vi "Update State Data.vi"(8 "error in (no error)":errorcluster, 9 "Data":variant, 10 "Argument":string, 11 "Window Action in":refnum<class "Window Action.lvclass">) -> (0 "error out":errorcluster, 3 "Window Action out":refnum<class "Window Action.lvclass">)   [LabVIEW 2020, in "MacroAssert.lvlib" / "Window Action.lvclass"]
uses:
  Window Action.lvclass
  Window Action Type.ctl
  Action Step/Action Step.lvclass
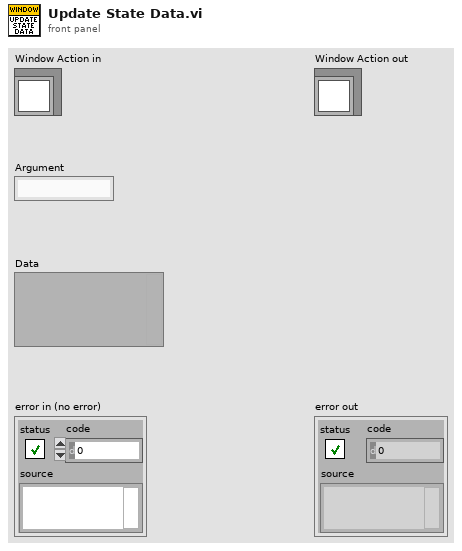
[diagram p1: front panel]
types:
  T1 = typedef "MacroAssert.lvlib/Window Action.lvclass/Window Action Type.ctl" = enum16{"Maximize Window", "Restore Window", "Minimize Window", "Close Window", "Bring Window to Front", "Send Window to Back"}
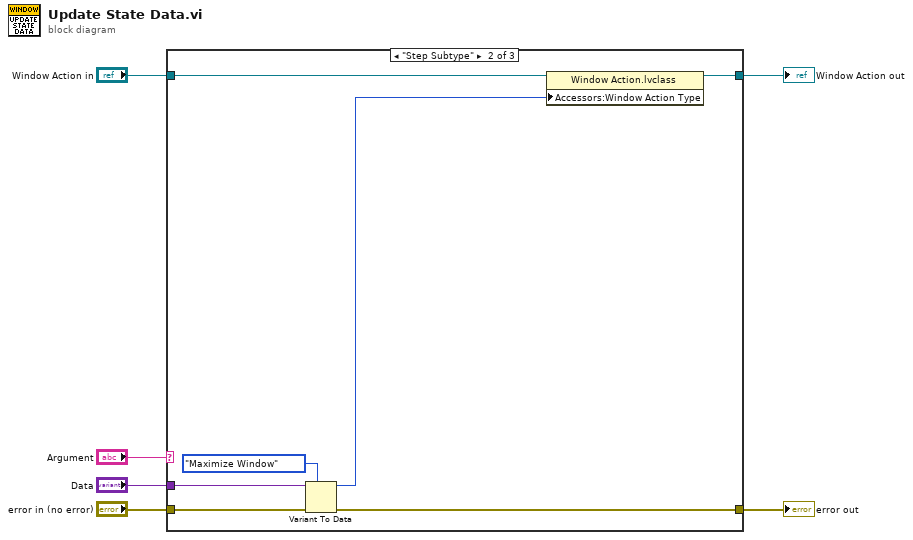
[diagram p0: block diagram]
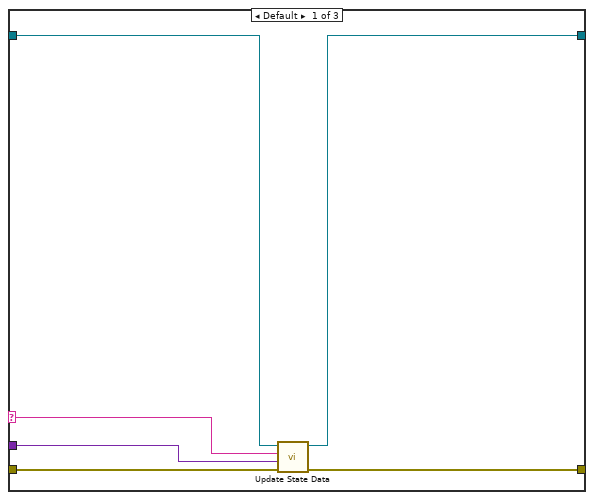
[diagram p2: hidden frame]
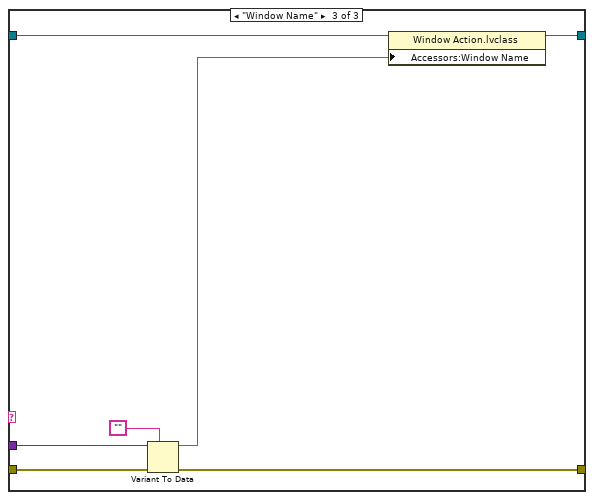
[diagram p3: hidden frame]
diagram:
  n1 = case shown="\"Step Subtype\"" "Argument" {
    selector: "Argument" -> [w9 _ _]
    tunnel: "Window Action in" -> [w8 w19 w26]
    tunnel: "error in (no error)" -> [w12 w17 w24]
    tunnel: [w7 w18 w25] -> w1
    tunnel: [w11 w16 w23] -> w6
    tunnel: "Data" -> [w10 w14 w22]
    frame Default {
      n2 = call-parent "Update State Data.vi"("error in (no error)"=w12, "Data"=w10, "Argument"=w9, "Step in"=w8) -> ("error out"=w11:errorcluster, "Step out"=w7:refnum<class "Window Action.lvclass">)  [unwired: 6 in]
    }
    frame "Step Subtype" {
      n3 = Variant To Data(error in=w17, type=Window_Action_Type."Maximize Window" ("Window Action Type"), Variant=w14) -> (data=w13:T1, error out=w16:errorcluster)
      n4 = property class="Window Action.lvclass"(reference=w19, "Accessors:Window Action Type"=w13) -> (reference out=w18:refnum<class "Window Action.lvclass">)  [unwired: 1 in, 1 out]
    }
    frame "Window Name" {
      n5 = Variant To Data(error in=w24, type="", Variant=w22) -> (data=w21:string, error out=w23:errorcluster)
      n6 = property class="Window Action.lvclass"(reference=w26, "Accessors:Window Name"=w21) -> (reference out=w25:refnum<class "Window Action.lvclass">)  [unwired: 1 in, 1 out]
    }
  }
  "error out" <- w6
  "Window Action out" <- w1
